vi "GetPosition.vi"(7 "Oriel (custom drivers) in":T1, 8 "error in (no error)":errorcluster) -> (0 "error out":errorcluster, 3 "Wavelength":dbl, 5 "Oriel (custom drivers) out":T1)   [LabVIEW 2017, in "Monochromator.lvlib" / "Oriel (custom drivers).lvlib"]
uses:
  Oriel (custom drivers).lvlib
  Controls/Params.ctl
  C:/Users/Abigail/Documents/Imperial Optical software/Optical Software Code Simplified/Modules/Monochromator/Cornerstone.dll
  Cornerstone.dll
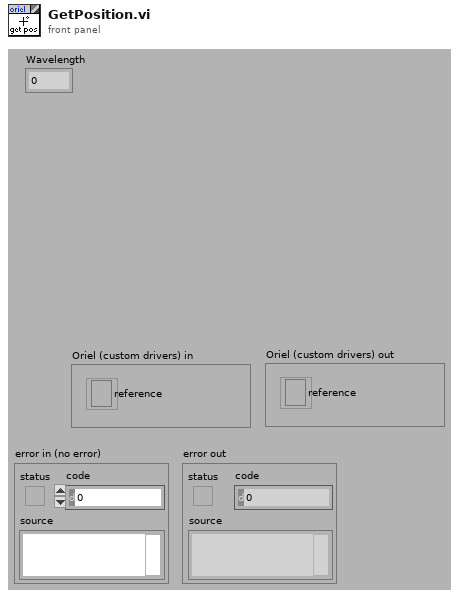
[diagram p1: front panel]
types:
  T1 = typedef "Monochromator.lvlib/Oriel (custom drivers).lvlib/Params.ctl" = cluster{"reference":refnum<k24>}
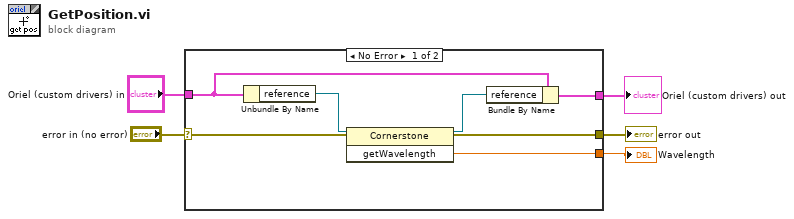
[diagram p0: block diagram]
diagram:
  n1 = case shown="No Error" "error in (no error)" {
    selector: "error in (no error)" -> [w12 w14]
    tunnel: [w11 w14] -> w4
    tunnel: [w10 w13] -> w3
    tunnel: "Oriel (custom drivers) in" -> [w7 w13]
    tunnel: [w6 _] -> w1
    frame No Error {
      n2 = Unbundle By Name(w7) -> ("reference"=w8:refnum<k24>)
      n3 = invoke class="Cornerstone" method="getWavelength"(reference=w8, error in=w12) -> (reference out=w9:refnum<k24>, error out=w11:errorcluster, "getWavelength"=w6:dbl)  [unwired: 1 in]
      n4 = Bundle By Name(cluster=w7, "reference"=w9) -> (w10:T1)
    }
    frame Error {
    }
  }
  "error out" <- w4
  "Oriel (custom drivers) out" <- w3
  "Wavelength" <- w1
